vi "remove class.vi"(7 "parent":refnum<class>, 8 "error in":errorcluster, 10 "child class":refnum<class>, 11 "refnum in":T1) -> (0 "error out":errorcluster, 3 "refnum out":T1)   [LabVIEW 2020, in "Publisher Subscriber.lvlib"]
uses:
  Publisher Subscriber.lvlib
  Controls/node refnum.ctl
  Controls/node dvr data.ctl
  Controls/data cluster.ctl
  Controls/subscription bank ref.ctl
  Controls/class dvr type.ctl
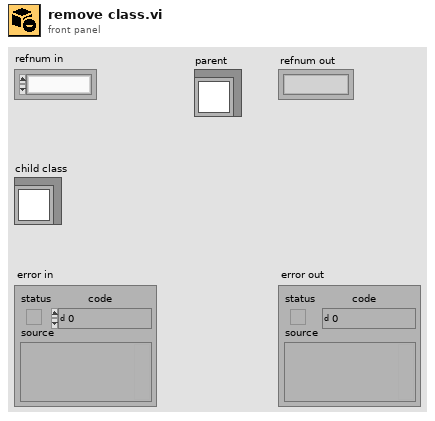
[diagram p1: front panel]
types:
  T1 = typedef "Publisher Subscriber.lvlib/node refnum.ctl" = refnum<k1>
  T2 = typedef "Publisher Subscriber.lvlib/node dvr data.ctl" = cluster{"queue ref":refnum<queue>, "Subscription Bank Ref":refnum<data-value>, "Command":string, "Data":variant, "Subscriptions []":set{string}, "Variables DVR Ref":refnum<data-value>}
  T3 = typedef "Publisher Subscriber.lvlib/class dvr type.ctl" = cluster{"Classes Map":map{string, refnum<class>}, "Name List[]":string[]}
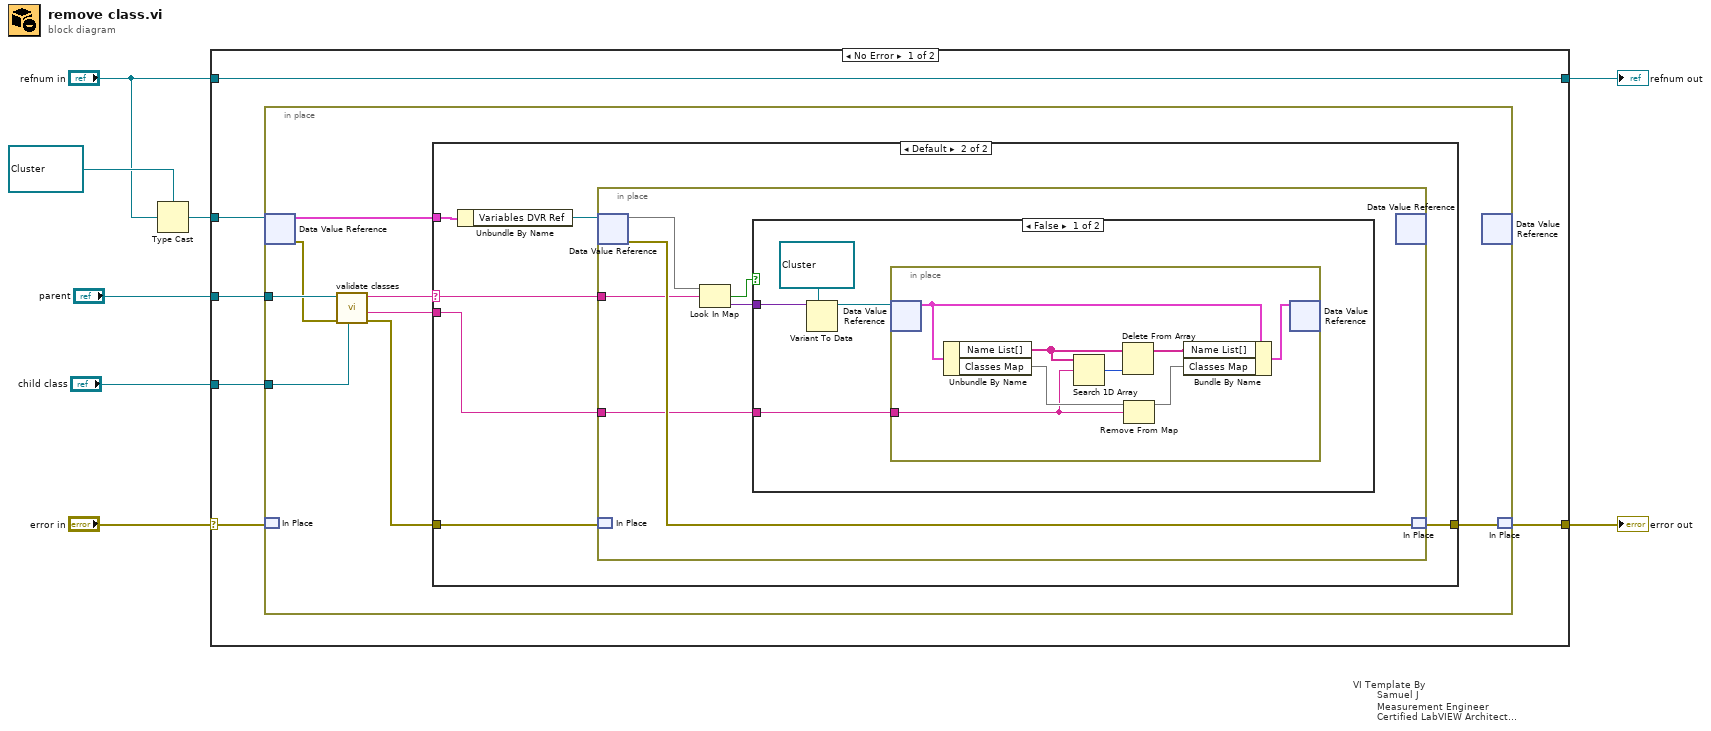
[diagram p0: block diagram]
diagram:
  n1 = Type Cast(type=refnum<data-value> refnum ("data value reference"), x="refnum in") -> (*(type *) &x=w5:refnum<data-value>)
  n2 = case "VI Template By\n        Samuel J\n        Measurement Engineer\n        Certified LabVIEW Architect\n        Vestas Technology R&D Chennai" shown="No Error" "error in" {
    selector: "error in" -> [w12 w49]
    tunnel: [w11 w49] -> w7
    tunnel: w5 -> [w13 _]
    tunnel: [w14 w48] -> w4
    tunnel: "refnum in" -> [w14 w48]
    tunnel: "parent" -> [w10 _]
    tunnel: "child class" -> [w9 _]
    frame No Error {
      n3 = in-place {
        in-place-border: w10 -> [w17]
        in-place-border: w9 -> [w20]
        n4 = in-place-dvr #1(w13) -> (w22:T2, w15:errorcluster)
        n5 = in-place-match #2(w12) -> ()  [unwired: 1 out]
        n6 = call "validate classes.vi"("Child"=w20, "error in"=w15, "Parent"=w17) -> ("error out"=w16:errorcluster, "class name"=w18:string, "unique parent name"=w19:string)  [unwired: 6 in]
        n7 = case shown="Default" w19 {
          selector: w19 -> [_ w24]
          tunnel: w22 -> [_ w29]
          tunnel: [w23 w27] -> w21
          tunnel: w16 -> [w23 w26]
          tunnel: w18 -> [_ w25]
          frame "" {
          }
          frame Default {
            n8 = Unbundle By Name(w29) -> ("Variables DVR Ref"=w28:refnum<data-value>)
            n9 = in-place {
              in-place-border: w24 -> [w31]
              in-place-border: w25 -> [w30]
              n10 = in-place-dvr #3(w28) -> (w34:map{string, variant}, w35:errorcluster)
              n11 = in-place-match #4(w26) -> ()  [unwired: 1 out]
              n12 = Look In Map(map=w34, key=w31) -> (key not found?=w32:bool, value=w33:variant)  [unwired: 1 in]
              n13 = case shown="False" w32 {
                tunnel: w33 -> [w39 _]
                tunnel: w30 -> [w36 _]
                frame False {
                  n14 = Variant To Data(type=refnum<data-value> refnum ("data value reference"), Variant=w39) -> (data=w37:refnum<data-value>)  [unwired: 1 in, 1 out]
                  n15 = in-place {
                    in-place-border: w36 -> [w41]
                    n16 = in-place-dvr #5(w37) -> (w47:T3)  [unwired: 1 out]
                    n17 = Unbundle By Name(w47) -> ("Name List[]"=w44:string[], "Classes Map"=w45:map{string, refnum<class>})
                    n18 = Search 1D Array(1D array=w44, element=w41) -> (index of element=w43:i32)  [unwired: 1 in]
                    n19 = Delete From Array(array=w44, index=w43) -> (array with subset deleted=w42:string[])  [unwired: 1 in, 1 out]
                    n20 = Remove From Map(10:w41, 11:w45) -> (3:w40:map{string, refnum<class>})  [unwired: 2 out]
                    n21 = Bundle By Name(cluster=w47, "Name List[]"=w42, "Classes Map"=w40) -> (w46:T3)
                    n22 = in-place-dvr #5(w46) -> ()  [unwired: 2 out]
                  }
                }
                frame True {
                }
              }
              n23 = in-place-dvr #3() -> ()  [unwired: 1 in, 2 out]
              n24 = in-place-match #4(w35) -> (w27:errorcluster)
            }
          }
        }
        n25 = in-place-dvr #1() -> ()  [unwired: 1 in, 2 out]
        n26 = in-place-match #2(w21) -> (w11:errorcluster)
      }
    }
    frame Error {
    }
  }
  "error out" <- w7
  "refnum out" <- w4
